vi "software_binning.vi"(1 "Bin image?":bool, 2 "Input Array":dbl[][](array[numeric])=[[1.0, 2.0, 3.0, 4.0, 5.0, 6.0, 1.0, 2.0], [7.0, 8.0, 9.0, 10.0, 11.0, 12.0, 4.0, 2.0], [13.0, 14.0, 15.0, 16.0, 17.0, 18.0, 60.0, 2.0], [19.0, 20.0, 21.0, 22.0, 23.0, 2.0, 10.0, 2.0], [25.0, 26.0, 27.0, 8.0, 29.0, 3.0, 6.0, 2.0], [31.0, 2.0, 33.0, 4.0, 35.0, 36.0, 5.0, 3.0], [4.0, 8.0, 0.0, 0.0, 0.0, 0.0, 7.0, 3.0], [5.0, 0.0, 0.0, 4.0, 5.0, 0.0, 2.0, 3.0], [50.0, 5.0, 0.0, 0.0, 20.0, 8.0, 5.0, 3.0], [3.0, 2.0, 400.0, 5.0, 10.0, 0.0, 4.0, 11.0], [8.0, 4.0, 5.0, 5.0, 7.0, 1.0, 1.0, 11.0], [4.0, 3.0, 1.0, 4.0, 42.0, 20.0, 8.0, 23.0]], 3 "bin size":i32=1) -> (0 "Binned Array":dbl[][](array[numeric]))   [LabVIEW 2013]
panel:
  out "SubArray - \npoints binned together":i32[][](array[numeric])
  out "Size of Input Array":i32[](array[numeric])
  out "Binned Image":dbl[][](graph)
  out "Uncut Image":dbl[][](graph)
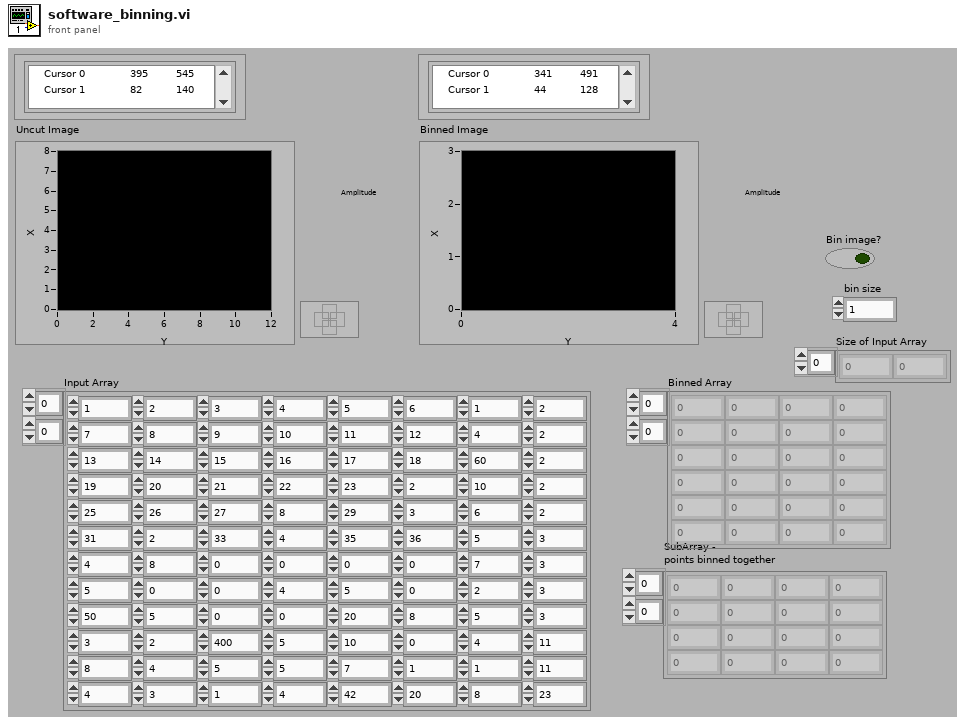
[diagram p1: front panel]
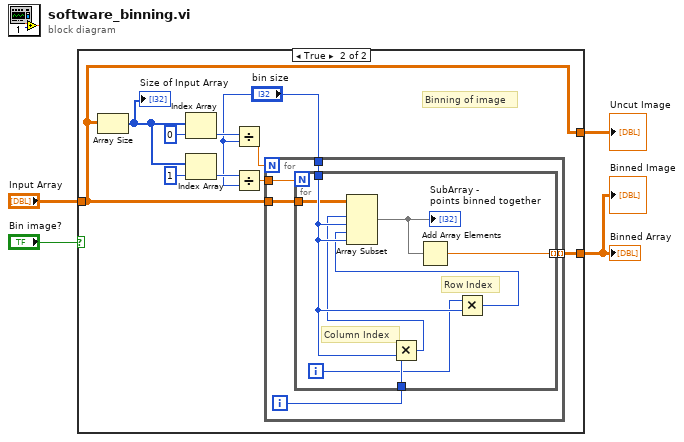
[diagram p0: block diagram]
diagram:
  n1 = case shown="True" "Bin image?" {
    tunnel: [w5 w7] -> w4
    tunnel: "Input Array" -> [w5 w6]
    tunnel: [w5 w6] -> w2
    frame False {
      # "No binning done.\nArray simply passed\nthrough."
    }
    frame True {
      # "Binning of image"
      n2 = Array Size(array=w6) -> (size(s)=w13:i32[])
      "Size of Input Array" <- w13
      n3 = Index Array(array=w13, index=0) -> (element=w11:i32)
      n4 = Index Array(array=w13, index=1) -> (element=w10:i32)
      n5 = Divide(x=w11, y="bin size") -> (x/y=w12:dbl)
      n6 = Divide(x=w10, y="bin size") -> (x/y=w9:dbl)
      n7 = for {
        N: w12 -> [_]
        tunnel: w6 -> [w19]
        tunnel: w9 -> [w20]
        tunnel: "bin size" -> [w18]
        tunnel: [w17] -> w7 mode=indexing
        i -> [w16]
        n8 = for {
          N: w20 -> [_]
          tunnel: w19 -> [w27]
          tunnel: w18 -> [w28]
          tunnel: w16 -> [w26]
          tunnel: [w25] -> w17 mode=indexing
          i -> [w24]
          # "Row Index"
          # "Column Index"
          n9 = Multiply(x=w26, y=w28) -> (x*y=w22:i32)
          n10 = Multiply(x=w24, y=w28) -> (x*y=w21:i32)
          n11 = Array Subset(array=w27, index (row)=w22, length (row)=w28, index (col)=w21, length (col)=w28) -> (w23:dbl[][])
          "SubArray - \npoints binned together" <- w23
          n12 = Add Array Elements(numeric array=w23) -> (sum=w25:dbl)
        }
      }
    }
  }
  "Binned Image" <- w4
  "Uncut Image" <- w2
  "Binned Array" <- w4
